vi "main.vi"() -> ()   [LabVIEW 2020]
panel:
  in  "y 2":dbl=5.0 format="%#_13g"
  out "x+y":dbl
  in  "y":dbl
  in  "x":dbl
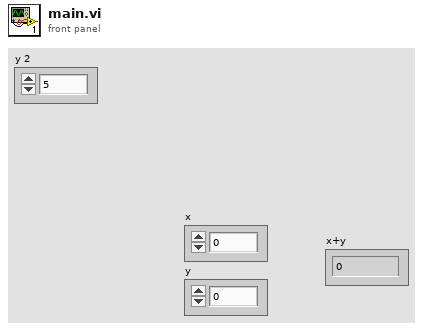
[diagram p1: front panel]
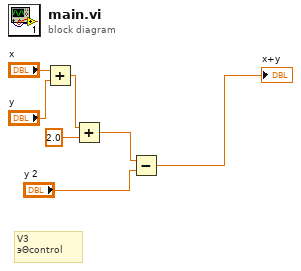
[diagram p0: block diagram]
diagram:
  # "V3\nэΘcontrol"
  n1 = Add(x="x", y="y") -> (x+y=w5:dbl)
  n2 = Add(x=w5, y=2.0) -> (x+y=w2:dbl)
  n3 = Subtract(x=w2, y="y 2") -> (x-y=→"x+y":dbl)
